vi "Populate_Tree.vi"(0 "Reference_In":refnum<vi>, 5 "File_Path":path, 7 "Parent_Tag":string, 11 "Error_In":errorcluster, 13 "Add_Parent_Too":bool) -> (4 "Reference_Out":refnum<vi>, 15 "Error_Out":errorcluster={"status"=FALSE, "code"=1088, "source"="Invoke Node in Untitled 1.vi:5370001->Untitled 1.vi:5370002->Untitled 1.vi:5370003->Untitled 1.vi\n<APPEND>\nMethod Name: <b>Edit Tree Items:Add Item</b>"})   [LabVIEW 2021]
doc: "Populate files into the tree"
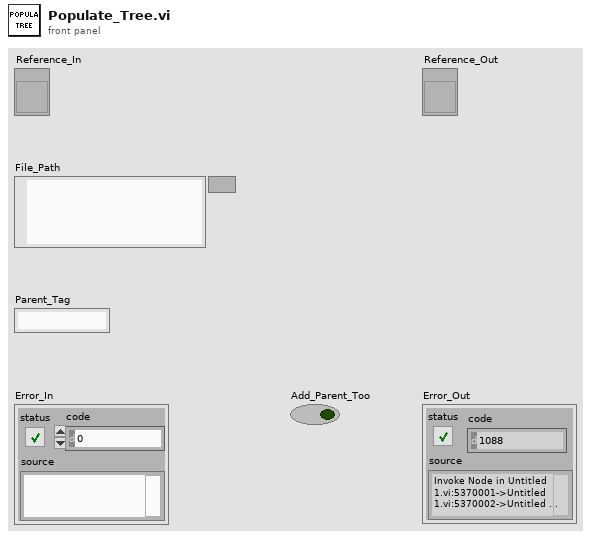
[diagram p1: front panel]
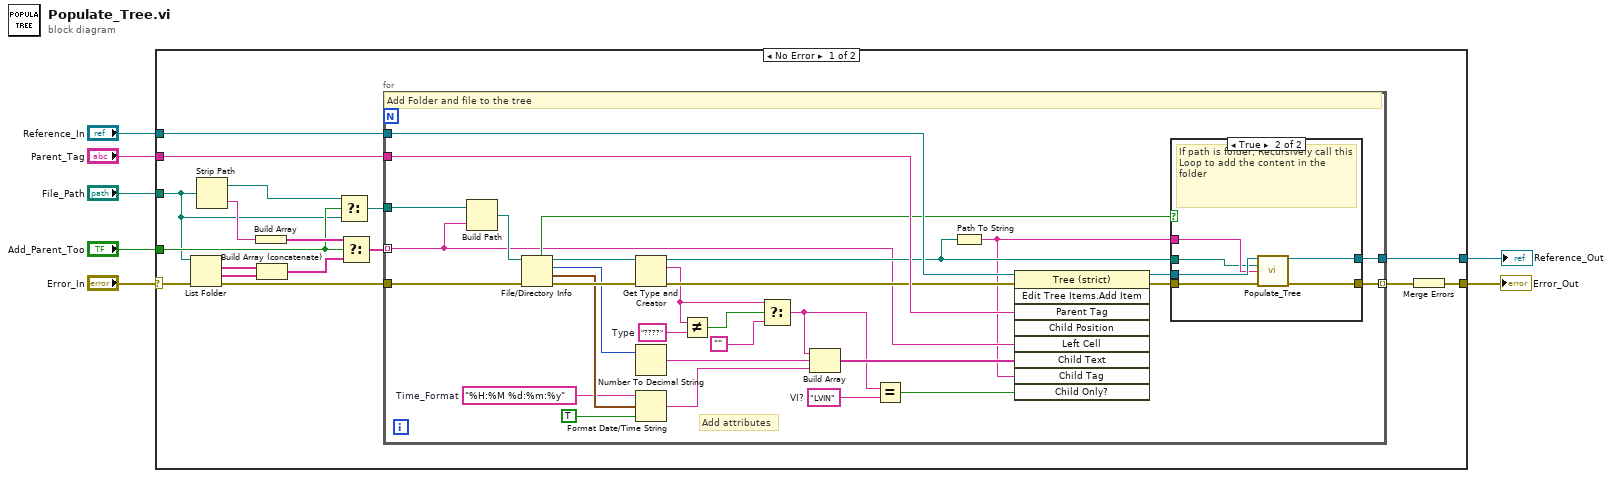
[diagram p0: block diagram]
diagram:
  n1 = case shown="No Error" "Error_In" {
    selector: "Error_In" -> [w16 w64]
    tunnel: "Parent_Tag" -> [w24 _]
    tunnel: "Reference_In" -> [w22 w63]
    tunnel: [w17 w64] -> w5
    tunnel: [w15 w63] -> w3
    tunnel: "Add_Parent_Too" -> [w9 _]
    tunnel: "File_Path" -> [w8 _]
    frame No Error {
      n2 = List Folder(path=w8, error in=w16) -> (filenames=w19:string[], folder names=w20:string[], error out=w21:errorcluster)  [unwired: 2 in, 1 out]
      n3 = Strip Path(path=w8) -> (stripped path=w14:path, name=w11:string)
      n4 = Build Array(w11) -> (w10:string[])
      n5 = Build Array (concatenate)(w19, w20) -> (w18:string[])
      n6 = Select(t=w14, s=w9, f=w8) -> (s? t:f=w13:path)
      n7 = Select(t=w10, s=w9, f=w18) -> (s? t:f=w12:string[])
      n8 = for {
        tunnel: w24 -> [w54]
        tunnel: [w53] -> w23 mode=indexing
        tunnel: w21 -> [w52]
        tunnel: w22 -> [w51]
        tunnel: w12 -> [w27] mode=indexing
        tunnel: w13 -> [w34]
        tunnel: [w30] -> w15
        w37 = "????"  # Type
        w40 = "LVIN"  # VI?
        w41 = "%H:%M %d:%m:%y"  # Time_Format
        # "Add attributes"
        # "Add Folder and file to the tree"
        n9 = Build Path(base path=w34, name or relative path=w27) -> (appended path=w29:path)
        n10 = File/Directory Info(path=w29, error in=w52) -> (path out=w49:path, directory=w31:bool, size=w46:i64, last mod=w45:timestamp, error out=w50:errorcluster)  [unwired: 2 out]
        n11 = Get Type and Creator(4:w50, 7:w49) -> (0:w48:errorcluster, 2:w38:string, 3:w28:path)  [unwired: 1 out]
        n12 = Number To Decimal String(number=w46) -> (decimal integer string=w44:string)  [unwired: 1 in]
        n13 = Format Date/Time String(time format string (%c)=w41, seconds (now)=w45, UTC format=TRUE) -> (date/time string=w43:string)
        n14 = Not Equal?(x=w38, y=w37) -> (x != y?=w36:bool)
        n15 = Select(t=w38, s=w36, f="") -> (s? t:f=w35:string)
        n16 = Build Array(w35, w44, w43) -> (w47:string[])
        n17 = Equal?(x=w35, y=w40) -> (x = y?=w25:bool)
        n18 = Path To String(path=w28) -> (string=w26:string)
        n19 = invoke on="Invoke Node" class="Tree (strict)" method="Edit Tree Items.Add Item"(reference=w51, error in=w48, "Parent Tag"=w54, "Left Cell"=w27, "Child Text"=w47, "Child Tag"=w26, "Child Only?"=w25) -> (reference out=w32:refnum<vi>, error out=w33:errorcluster)  [unwired: 2 in, 7 out]
        n20 = case shown="True" w31 {
          tunnel: [w56 w62] -> w53
          tunnel: w33 -> [w56 w61]
          tunnel: w32 -> [w55 w60]
          tunnel: w28 -> [_ w58]
          tunnel: w26 -> [_ w59]
          tunnel: [w55 w57] -> w30
          frame False {
          }
          frame True {
            # "If path is folder, Recursively call this Loop to add the content in the folder"
            n21 = call "Populate_Tree.vi"("Reference_In"=w60, "File_Path"=w58, "Parent_Tag"=w59, "Error_In"=w61) -> ("Reference_Out"=w57:refnum<vi>, "Error_Out"=w62:errorcluster)  [unwired: 10 in]
          }
        }
      }
      n22 = Merge Errors(w23) -> (w17:errorcluster)
    }
    frame Error {
    }
  }
  "Error_Out" <- w5
  "Reference_Out" <- w3
